vi "Get NF Frequency.vi"(8 "error in (no error)":errorcluster, 11 "NF in":refnum<class "NF.lvclass">) -> (0 "error out":errorcluster, 2 "NF frequency":string, 3 "NF out":refnum<class "NF.lvclass">)   [LabVIEW 2018, in "NF.lvlib" / "NF.lvclass"]
uses:
  NF.lvclass
  C:/Sequence Automation/Plugins/Measurement Interface.lvlibp/Measurement Interface.lvclass
  Plugins/Measurement Interface.lvlibp/Private Methods/Measurement Parameters/Read Measurement Parameters.vi
  Plugins/String Database.lvlibp/String Database.lvclass
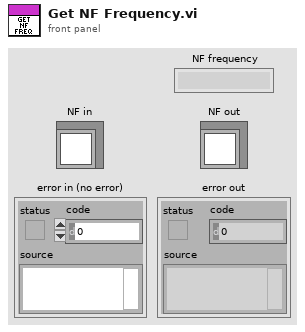
[diagram p1: front panel]
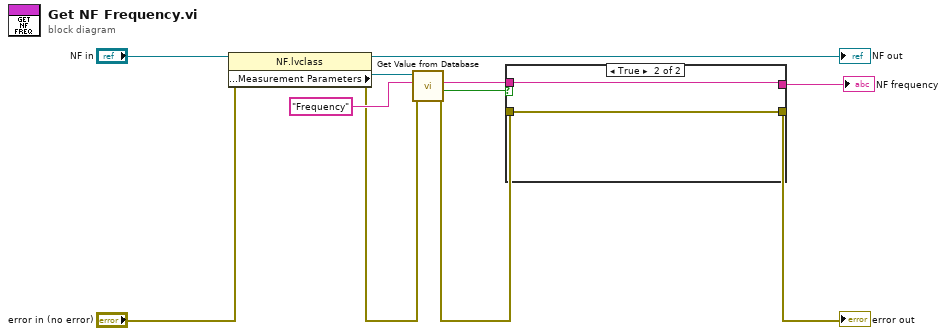
[diagram p0: block diagram]
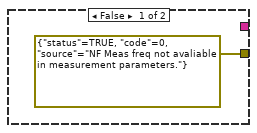
[diagram p2: hidden frame]
diagram:
  n1 = property class="NF.lvclass"(reference="NF in", error in="error in (no error)") -> (reference out=→"NF out":refnum<class "NF.lvclass">, error out=w6:errorcluster, "Protected Methods:Measurement Parameters"=w8:refnum<class "String Database.lvclass">)
  n2 = call "Get Value from Database.vi"("error in (no error)"=w6, "Entry Name"="Frequency", "Message in"=w8) -> ("error out"=w4:errorcluster, "Entry Found"=w5:bool, "Entry Value"=w2:string)  [unwired: 5 in, 1 out]
  n3 = case shown="True" w5 {
    tunnel: w4 -> [_ w13]
    tunnel: [errorcluster {"status"=TRUE, "code"=0, "source"="NF Meas freq not avaliable in measurement parameters."} ("error out") w13] -> w3
    tunnel: w2 -> [_ w14]
    tunnel: [_ w14] -> w1
    frame False {
    }
    frame True {
    }
  }
  "error out" <- w3
  "NF frequency" <- w1
